vi "CreatePublicEvents.vi"(8 "error in (no error)":errorcluster, 11 "SMO.TimedLoop":refnum<class "SMO.TimedLoop.lvclass">) -> (0 "error out":errorcluster, 3 "SMO.TimedLoop out":refnum<class "SMO.TimedLoop.lvclass">)   [LabVIEW 2013, in "SMO.TimedLoop.lvclass"]
doc: "---------------------------------------------------------------\nJKI State Machine Objects™\nhttp://jki.net/state-machine-objects/\nCopyright (C) 2005-2015, JKI <info@jki.net>\nALL RIGHTS RESERVEDJKI State Machine Objects (SMO) 1.0.0.5\nJKI - JKI\nCopyright (c) 2016, JKI"
uses:
  SMO.TimedLoop.lvclass
  Typedefs/SetpointChanged--EventData--Cluster.ctl
  Typedefs/Data.ctl
  <vilib>/JKI/JKI SMO/SMO/SMO.lvclass
  SMO.TimedLoop.lvclass/SMO.TimedLoop.ctl
panel:
  # "For instructions on how to use the JKI State Machine Objects, examples and video tutorials, visit:\nhttp://jki.net/state-machine-objects/\n\nJKI State Machine Objects™\nhttp://jki.net/state-machine-objects/\nCopyright (C) 2005-2015, JKI <info@jki.net>\nALL RIGHTS RESERVED"
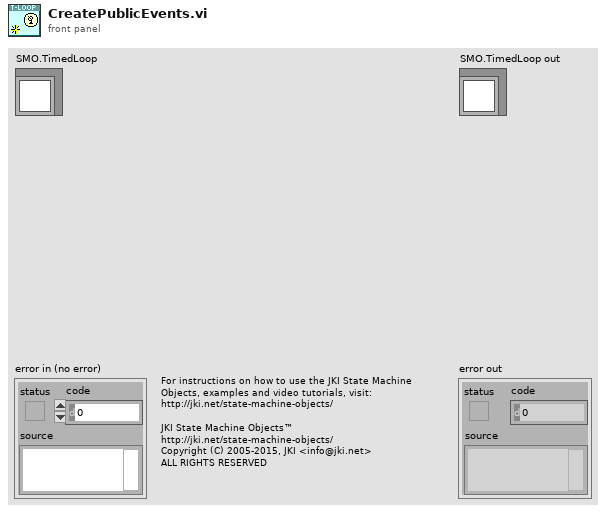
[diagram p1: front panel]
types:
  T1 = typedef "SMO.TimedLoop.lvclass/Data.ctl" = dbl
  T2 = typedef "SMO.TimedLoop.lvclass/SetpointChanged--EventData--Cluster.ctl" = cluster{"Setpoint":T1}
  T3 = typedef "SMO.TimedLoop.lvclass/PrivateData--Ref.ctl" = refnum<data-value>
  T4 = typedef "SMO.TimedLoop.lvclass/PrivateData--Cluster.ctl" = cluster{"Public Events":T5, "Setpoint":T1, "Private Events":T6}
  T5 = typedef "SMO.TimedLoop.lvclass/PublicEvents--Cluster.ctl" = cluster{"Setpoint Changed":refnum<user-event>, "Value Changed":refnum<user-event>}
  T6 = typedef "SMO.TimedLoop.lvclass/PrivateEvents--Cluster.ctl" = cluster{"AsyncMethod":refnum<user-event>}
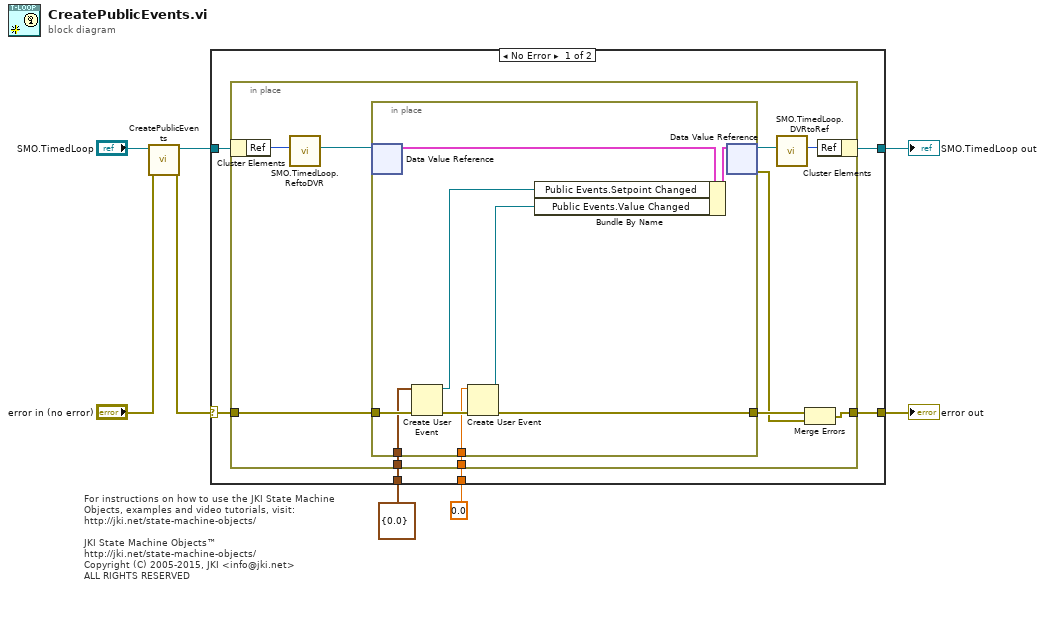
[diagram p0: block diagram]
diagram:
  # "For instructions on how to use the JKI State Machine Objects, examples and video tutorials, visit:\nhttp://jki.net/state-machine-objects/\n\nJKI State Machine Objects™\nhttp://jki.net/state-machine-objects/\nCopyright (C) 2005-2015, JKI <info@jki.net>\nALL RIGHTS RESERVED"
  n1 = call-parent "CreatePublicEvents.vi"("error in (no error)"="error in (no error)", "SMO"="SMO.TimedLoop") -> ("error out"=w2:errorcluster, "SMO out"=w4:refnum<class "SMO.TimedLoop.lvclass">)  [unwired: 8 in]
  n2 = case shown="No Error" w2 {
    selector: w2 -> [w12 w35]
    tunnel: [w11 w35] -> w7
    tunnel: [w13 w34] -> w8
    tunnel: w4 -> [w14 w34]
    tunnel: T2 {"Setpoint"=0.0} ("Data In Event Data") -> [w10 _]
    tunnel: T1 0.0 ("Data") -> [w9 _]
    frame No Error {
      n3 = in-place {
        in-place-border: w12 -> [w24]
        in-place-border: [w21] -> w11
        in-place-border: w10 -> [w20]
        in-place-border: w9 -> [w15]
        n4 = in-place-cluster #1(w14) -> ("Ref"=w19:u32)
        n5 = call "SMO.TimedLoop.ReftoDVR.vi"("Ref"=w19) -> ("Ref"=w18:T3)  [unwired: 10 in]
        n6 = in-place {
          in-place-border: w24 -> [w31]
          in-place-border: [w27] -> w23
          in-place-border: w20 -> [w30]
          in-place-border: w15 -> [w26]
          n7 = in-place-dvr #2(w18) -> (w32:T4)  [unwired: 1 out]
          n8 = Create User Event(user event datatype=w30, error in=w31) -> (user event=w29:refnum<user-event>, error out=w28:errorcluster)
          n9 = Create User Event(user event datatype=w26, error in=w28) -> (user event=w25:refnum<user-event>, error out=w27:errorcluster)
          n10 = Bundle By Name(cluster=w32, "Public Events.Setpoint Changed"=w29, "Public Events.Value Changed"=w25) -> (w33:T4)
          n11 = in-place-dvr #2(w33) -> (w17:T3, w22:errorcluster)
        }
        n12 = call "SMO.TimedLoop.DVRtoRef.vi"("Ref"=w17) -> ("Ref"=w16:u32)  [unwired: 10 in]
        n13 = Merge Errors(w23, w22) -> (w21:errorcluster)
        n14 = in-place-cluster #1("Ref"=w16) -> (w13:refnum<class "SMO.TimedLoop.lvclass">)
      }
    }
    frame Error {
    }
  }
  "error out" <- w7
  "SMO.TimedLoop out" <- w8
